vi "ui folder size tree.vi"() -> ()   [LabVIEW 2023]
panel:
  out "size(s)":i32
  out "string":string
  in  "folder depth":i32=-1
  in  "Folder Path":path
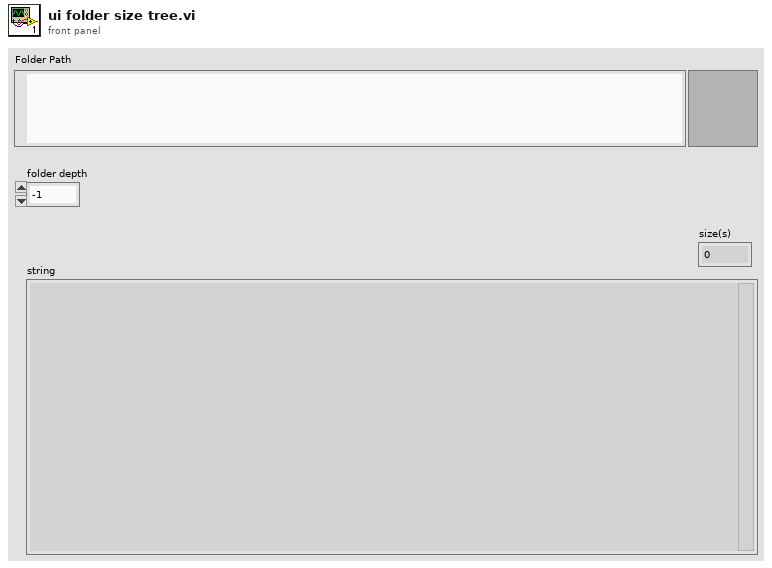
[diagram p1: front panel]
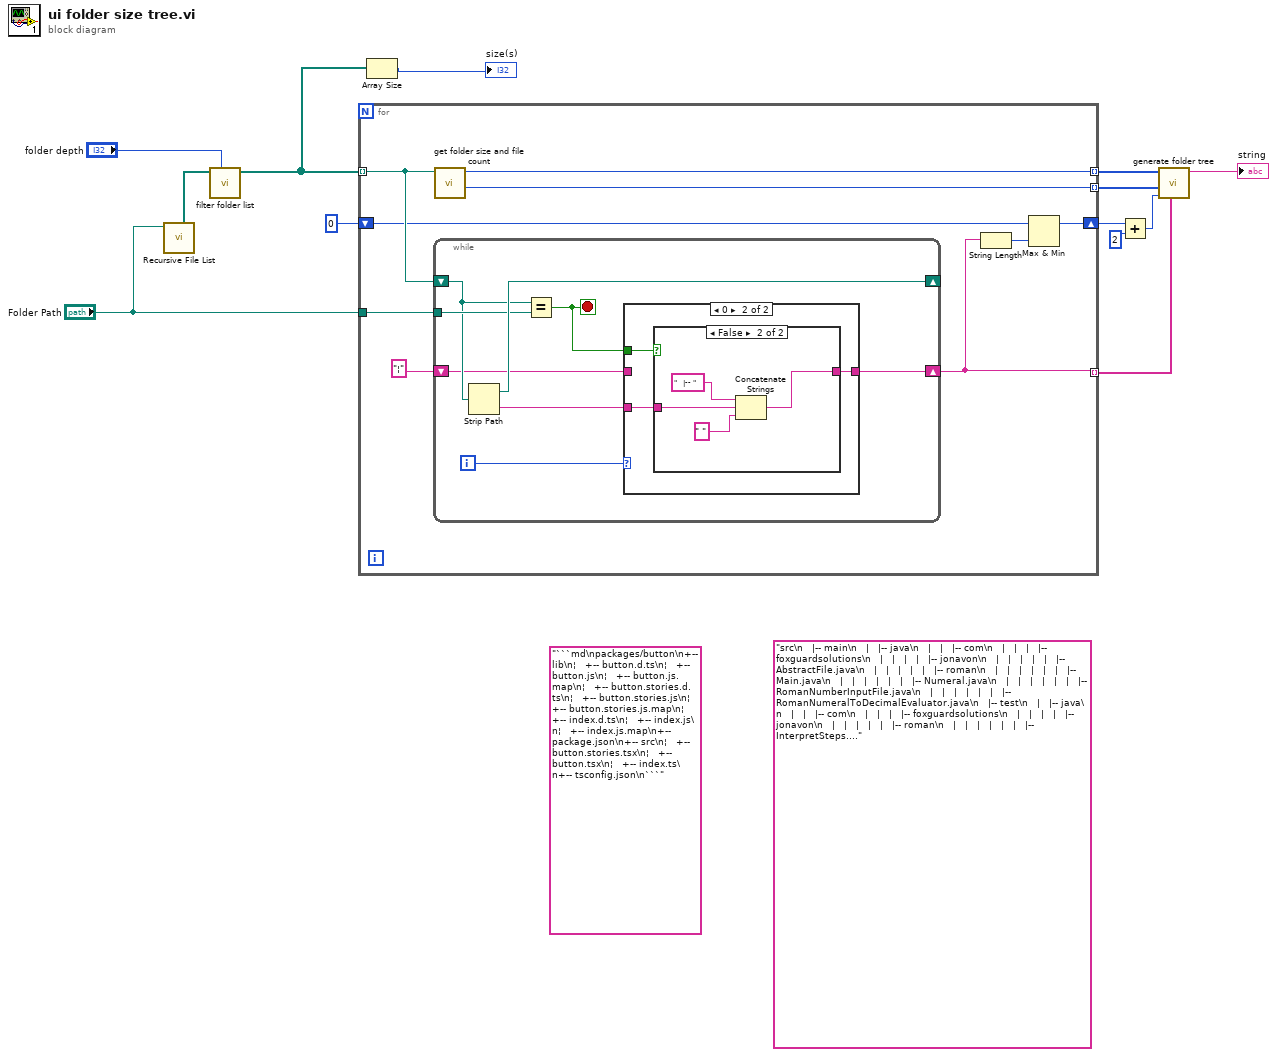
[diagram p0: block diagram]
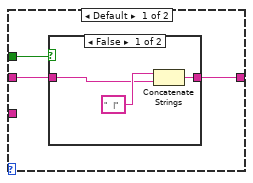
[diagram p2: hidden frame]
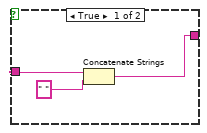
[diagram p4: hidden frame]
diagram:
  (unwired) "src\n   |-- main\n   |   |-- java\n   |   |   |-- com\n   |   |   |   |-- foxguardsolutions\n   |   |   |   |   |-- jonavon\n   |   |   |   |   |   |-- AbstractFile.java\n   |   |   |   |   |   |-- roman\n   |   |   |   |   |   |   |-- Main.java\n   |   |   |   |   |   |   |-- Numeral.java\n   |   |   |   |   |   |   |-- RomanNumberInputFile.java\n   |   |   |   |   |   |   |-- RomanNumeralToDecimalEvaluator.java\n   |-- test\n   |   |-- java\n   |   |   |-- com\n   |   |   |   |-- foxguardsolutions\n   |   |   |   |   |-- jonavon\n   |   |   |   |   |   |-- roman\n   |   |   |   |   |   |   |-- InterpretSteps.java\n   |   |   |   |   |   |   |-- RunCukesTest.java\n   |   |-- resources\n   |   |   |-- com\n   |   |   |   |-- foxguardsolutions\n   |   |   |   |   |-- jonavon\n   |   |   |   |   |   |-- roman\n   |   |   |   |   |   |   |-- Interpret.feature\n   |   |   |-- sample-input.txt"
  (unwired) "```md\npackages/button\n+-- lib\n¦   +-- button.d.ts\n¦   +-- button.js\n¦   +-- button.js.map\n¦   +-- button.stories.d.ts\n¦   +-- button.stories.js\n¦   +-- button.stories.js.map\n¦   +-- index.d.ts\n¦   +-- index.js\n¦   +-- index.js.map\n+-- package.json\n+-- src\n¦   +-- button.stories.tsx\n¦   +-- button.tsx\n¦   +-- index.ts\n+-- tsconfig.json\n```"
  n1 = call <vilib>:"Recursive File List.vi"("Folder Path"="Folder Path") -> ("All Folders"=w12:path[])  [unwired: 6 in, 4 out]
  n2 = call "filter folder list.vi"("folder depth"="folder depth", "All Folders"=w12) -> ("All Folders 2"=w2:path[])  [unwired: 8 in, 1 out]
  n3 = for {
    tunnel: w2 -> [w20] mode=indexing
    tunnel: "Folder Path" -> [w22]
    tunnel: [w19] -> w9 mode=indexing
    tunnel: [w14] -> w8 mode=indexing
    tunnel: [w18] -> w6 mode=indexing
    shift-right: [w15] -> w7
    shift-left: 0 -> [w16]
    n4 = while {
      tunnel: w22 -> [w27]
      shift-right: [w28] -> _
      shift-left: w20 -> [w25]
      shift-right: [w29] -> w18
      shift-left: "¦" ("string") -> [w23]
      i -> [w30]
      stop <- w24 stop-if-true
      n5 = Strip Path(path=w25) -> (stripped path=w28:path, name=w26:string)
      n6 = Equal?(x=w25, y=w27) -> (x = y?=w24:bool)
      n7 = case shown="0" w30 {
        tunnel: [w32 w40] -> w29
        tunnel: w24 -> [w31 w38]
        tunnel: w26 -> [_ w39]
        tunnel: w23 -> [w33 _]
        frame Default {
          n8 = case shown="False" w31 {
            tunnel: w33 -> [w35 w37]
            tunnel: [w34 w37] -> w32
            frame False {
              n9 = Concatenate Strings("   |" ("f"), w35) -> (w34:string)
            }
            frame True {
            }
          }
        }
        frame 0 {
          n10 = case shown="False" w38 {
            tunnel: [w43 w46] -> w40
            tunnel: w39 -> [w42 w45]
            frame True {
              n11 = Concatenate Strings(w42, " " ("string")) -> (w43:string)
            }
            frame False {
              n12 = Concatenate Strings("   |-- " ("f"), w45, " " ("string")) -> (w46:string)
            }
          }
        }
      }
    }
    n13 = call "get folder size and file count.vi"("Path"=w20) -> ("Number of Files"=w14:i32, "size"=w19:i64)  [unwired: 9 in]
    n14 = String Length(string=w18) -> (length=w17:i32)
    n15 = Max & Min(x=w16, y=w17) -> (max(x,y)=w15:i32)  [unwired: 1 out]
  }
  n16 = Array Size(array=w2) -> (size(s)=→"size(s)":i32)
  n17 = Add(x=w7, y=2 ("x")) -> (x+y=w4:i32)
  n18 = call "generate folder tree.vi"("folder names[]"=w6, "max length"=w4, "file count"=w8, "Size"=w9) -> ("string"=→"string":string)  [unwired: 7 in]
